vi "Case_Enum.vi"() -> ()   [LabVIEW 2016]
panel:
  in  "Enum":T1(ring)
  out "Numeric Indicator":dbl
  in  "B":dbl
  in  "A":dbl
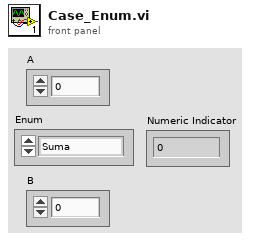
[diagram p1: front panel]
types:
  T1 = enum16{"Suma", "Resta", "Multiplicacion", "Division"}
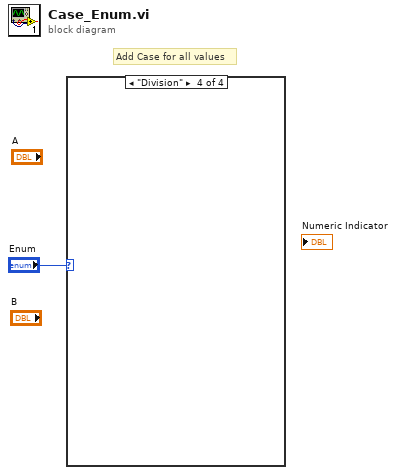
[diagram p0: block diagram]
diagram:
  # "Add Case for all values"
  n1 = case shown="\"Division\"" "Enum" {
    frame "Suma", Default {
    }
    frame "Resta" {
    }
    frame "Multiplicacion" {
    }
    frame "Division" {
    }
  }
